vi "Check SDK Installed.vi"(8 "error in":errorcluster) -> (0 "error out":errorcluster, 3 ".Net SDK Available?":bool)   [LabVIEW 2026]
panel:
  out "Available .NET SDKs":dbl[](array[numeric])
  out "standard output":string
  out "standard error":string
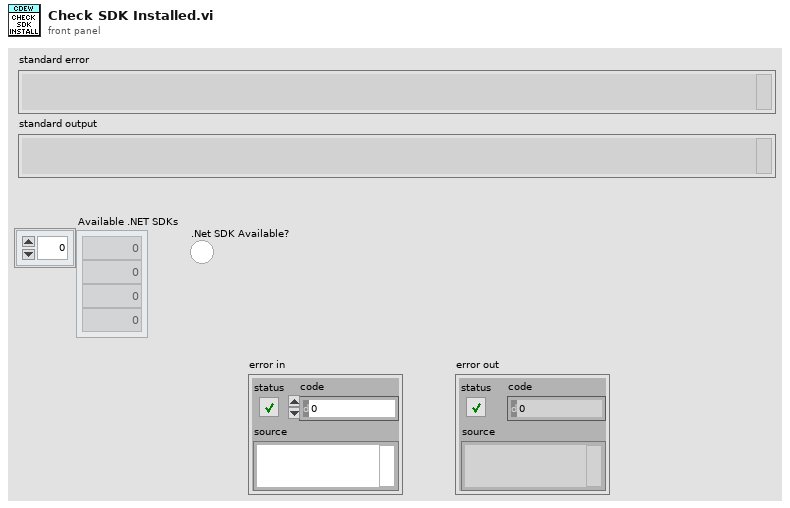
[diagram p1: front panel]
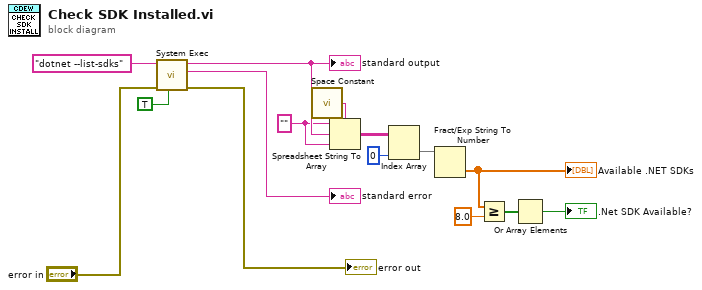
[diagram p0: block diagram]
diagram:
  w11 = "" ("format string")
  n1 = call <vilib>:"System Exec.vi"("run minimized? (F)"=TRUE, "error in (no error)"="error in", "command line"="dotnet --list-sdks") -> ("error out"=→"error out":errorcluster, "standard error"=→"standard error":string, "standard output"=w13:string)  [unwired: 5 in, 1 out]
  "standard output" <- w13
  n2 = call <vilib>:"Space Constant.vi"() -> ("String"=w12:string)
  n3 = Spreadsheet String To Array(delimiter (Tab)=w12, format string=w11, spreadsheet string=w13, array type (2D Dbl)=w11) -> (array=w9:string[][])
  n4 = Index Array(array=w9, index (col)=0) -> (element=w7:string[])  [unwired: 1 in]
  n5 = Fract/Exp String To Number(string=w7) -> (number=w6:dbl[])  [unwired: 3 in, 1 out]
  "Available .NET SDKs" <- w6
  n6 = Greater Or Equal?(x=w6, y=8.0) -> (x >= y?=w4:bool[])
  n7 = Or Array Elements(Boolean array=w4) -> (logical OR=→".Net SDK Available?":bool)
